vi "Fully Custom Page.vi"(8 "error in (no error)":errorcluster, 11 "Node Ptr":T2 format="%.0x") -> (0 "error out":errorcluster)   [LabVIEW 2011, in "Engine Sim System Explorer.lvlib"]
uses:
  Engine Sim System Explorer.lvlib
  <vilib>/NI Veristand/Custom Device API/Custom Device Item Ref.ctl
  TypeDefs/AngleReference.ctl
  Shared/Engine Simulation Global.vi
  <vilib>/NI Veristand/Custom Device API/Get Item Property (Boolean).vi
  <vilib>/NI Veristand/Custom Device API/Get Item Property (Variant).vi
  <vilib>/NI Veristand/Custom Device API/Get Item Property (U16).vi
  <vilib>/NI Veristand/Custom Device API/Set Item Property (Variant).vi
  <vilib>/NI Veristand/Custom Device API/Set Item Property (Boolean).vi
  <vilib>/Utility/file.llb/Read From Spreadsheet File (DBL).vi
  <vilib>/Utility/file.llb/Write To Spreadsheet File (DBL).vi
  <vilib>/NI Veristand/Custom Device API/Custom Device API.lvlib
  Engine Simulation Shared.lvlib
panel:
  in  "CycleAngle?":T1=TRUE caption="FPGA Simulation Angle Reference"
  in  "Export":bool
  in  "Import":bool
  in  "Tooth Angles":cluster{"Falling Edge":dbl, "Rising Edge":dbl}[](array[cluster])
  in  "SHDocVw.IWebBrowser2":refnum<k7>(container)
  out "N Teeth M Missing View":picture
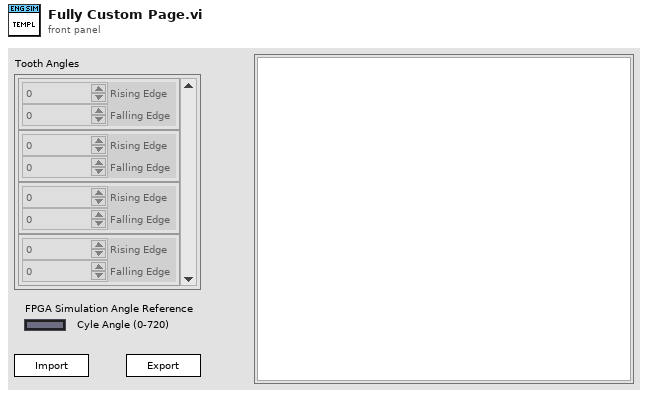
[diagram p1: front panel]
types:
  T1 = typedef "Engine Sim System Explorer.lvlib/AngleReference.ctl" = bool
  T2 = typedef "Custom Device API.lvlib/Custom Device Item Ref.ctl" = u64
  T3 = typedef "Custom Device API.lvlib/Custom Device Commands.ctl" = enum16{"Default", "Item renamed", "Shutdown", "Dynamic button pressed"}
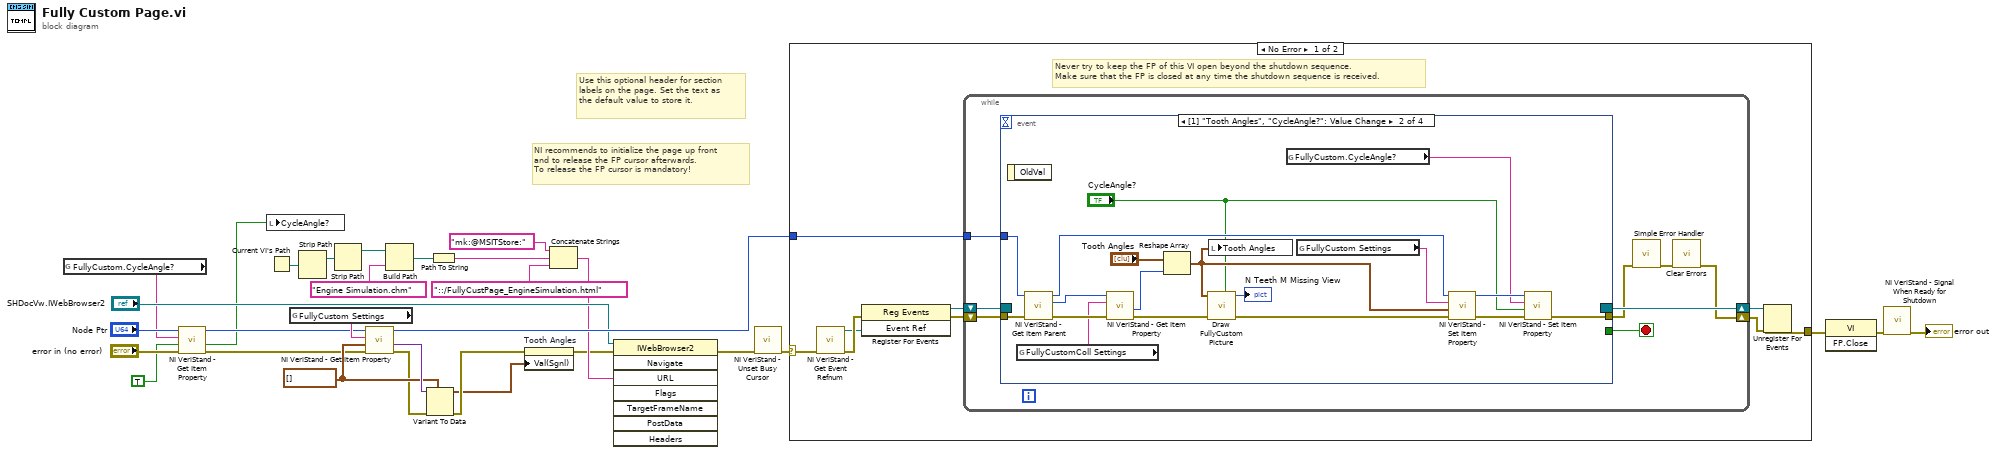
[diagram p0: block diagram]
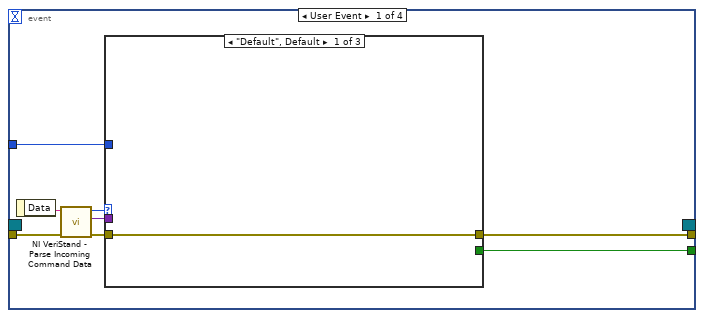
[diagram p2: hidden frame]
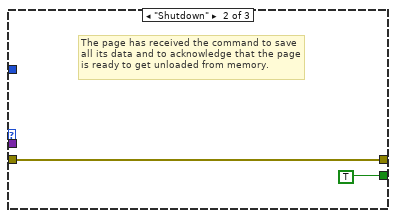
[diagram p3: hidden frame]
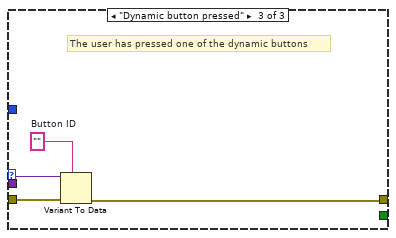
[diagram p4: hidden frame]
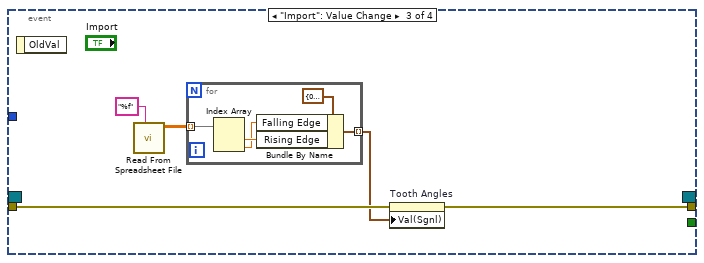
[diagram p5: hidden frame]
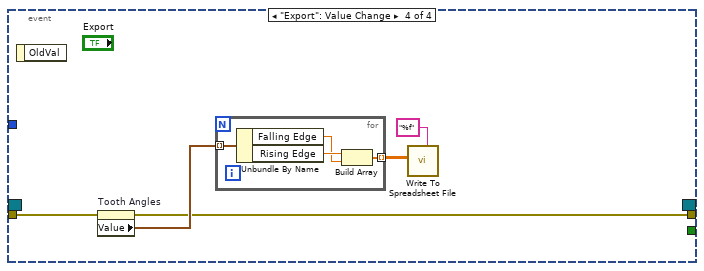
[diagram p6: hidden frame]
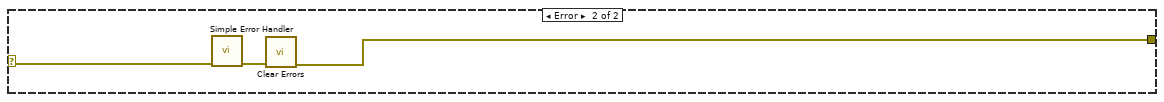
[diagram p7: hidden frame]
diagram:
  w11 = cluster{"Falling Edge":dbl, "Rising Edge":dbl}[] [] ("Tooth Angles")
  # "Use this optional header for section labels on the page. Set the text as the default value to store it."
  # "NI recommends to initialize the page up front\nand to release the FP cursor afterwards.\nTo release the FP cursor is mandatory!"
  n1 = global read "Engine Simulation Global.vi" "FullyCustom.CycleAngle?"() -> (w5:string)
  n2 = call-poly <vilib>:"NI VeriStand - Get Item Property.vi"("error in (no error)"="error in (no error)", "Default Value"=TRUE, "Property Name"=w5, "Item Ref in"="Node Ptr") -> ("error out"=w2:errorcluster, "Value"=w1:bool, "Item Ref out"=w3:T2)  [unwired: 4 in, 1 out]
  n3 = local write "CycleAngle?"(w1) -> ()
  n4 = Current VI's Path() -> (path=w22:path)
  n5 = global read "Engine Simulation Global.vi" "FullyCustom Settings"() -> (w13:string)
  n6 = Strip Path(path=w22) -> (stripped path=w21:path)  [unwired: 1 out]
  n7 = Strip Path(path=w21) -> (stripped path=w16:path)  [unwired: 1 out]
  n8 = call-poly <vilib>:"NI VeriStand - Get Item Property.vi"("error in (no error)"=w2, "Default Value"=w11, "Property Name"=w13, "Item Ref in"=w3) -> ("error out"=w10:errorcluster, "Value"=w12:variant, "Item Ref out"=w25:T2)  [unwired: 4 in, 1 out]
  n9 = Build Path(base path=w16, name or relative path="Engine Simulation.chm") -> (appended path=w18:path)
  n10 = Variant To Data(error in=w10, type=w11, Variant=w12) -> (data=w8:cluster{"Falling Edge":dbl, "Rising Edge":dbl}[], error out=w9:errorcluster)
  n11 = Path To String(path=w18) -> (string=w19:string)
  n12 = property on="Tooth Angles" class="Arr (strict)"(error in=w9, "Val(Sgnl)"=w8) -> (error out=w14:errorcluster)  [unwired: 1 in, 1 out]
  n13 = Concatenate Strings("mk:@MSITStore:" ("string"), w19, "::/FullyCustPage_EngineSimulation.html" ("name or relative path")) -> (w15:string)
  n14 = invoke class="IWebBrowser2" method="Navigate"(reference="SHDocVw.IWebBrowser2", error in=w14, "URL"=w15) -> (error out=w27:errorcluster)  [unwired: 5 in, 7 out]
  n15 = call <vilib>:"NI VeriStand - Unset Busy Cursor.vi"("error in (no error)"=w27) -> ("error out"=w26:errorcluster)  [unwired: 10 out]
  n16 = case shown="No Error" w26 {
    selector: w26 -> [w31 w102]
    tunnel: [w36 w100] -> w30
    tunnel: w25 -> [w32 _]
    frame No Error {
      # "Never try to keep the FP of this VI open beyond the shutdown sequence.\nMake sure that the FP is closed at any time the shutdown sequence is received."
      n17 = call <vilib>:"NI VeriStand - Get Event Refnum.vi"("error in (no error)"=w31) -> ("error out"=w39:errorcluster, "Event Ref"=w35:refnum<user-event>)  [unwired: 9 out]
      n18 = register-events(error in=w39, w35) -> (reference out=w33:refnum<event-registration>, error out=w34:errorcluster)  [unwired: 1 in]
      n19 = while {
        tunnel: w32 -> [w43]
        shift-right: [w40] -> w37
        shift-left: w34 -> [w46]
        shift-right: [w47] -> w38
        shift-left: w33 -> [w45]
        stop <- w44 stop-if-true
        n20 = event shown="[1] \"Tooth Angles\", \"CycleAngle?\": Value Change" {
          selector: w45 -> [_ _ _ _]
          dyn-events: [_ _ _ _] -> w47
          timeout: _ -> [_ _ _ _]
          tunnel: w46 -> [w55 w75 w83 w95]
          tunnel: [w51 _ _ _] -> w44
          tunnel: [w50 w65 w82 w93] -> w42
          tunnel: w43 -> [w49 w74 _ _]
          event User Event {
            n21 = event-data() -> ("Data"=w54:string)  [unwired: 1 out]
            n22 = call <vilib>:"NI VeriStand - Parse Incoming Command Data.vi"("error in (no error)"=w55, "Incoming data"=w54) -> ("error out"=w53:errorcluster, "Outgoing data"=w48:variant, "Action"=w52:T3)  [unwired: 7 out]
            n23 = case shown="\"Default\", Default" w52 {
              tunnel: w53 -> [w56 w57 w62]
              tunnel: [_ TRUE _] -> w51
              tunnel: [w56 w57 w59] -> w50
              tunnel: w49 -> [_ _ _]
              tunnel: w48 -> [_ _ w61]
              frame "Default", Default {
              }
              frame "Shutdown" {
                # "The page has received the command to save all its data and to acknowledge that the page is ready to get unloaded from memory."
              }
              frame "Dynamic button pressed" {
                w60 = ""  # Button ID
                # "The user has pressed one of the dynamic buttons"
                n24 = Variant To Data(error in=w62, type=w60, Variant=w61) -> (error out=w59:errorcluster)  [unwired: 1 out]
              }
            }
          }
          event "Tooth Angles": Value Change {
            n25 = event-data() -> ()  [unwired: 2 out]
            n26 = global read "Engine Simulation Global.vi" "FullyCustomColl Settings"() -> (w69:string)
            n27 = call <vilib>:"NI VeriStand - Get Item Parent.vi"("error in (no error)"=w75, "Item Ref in"=w74) -> ("error out"=w72:errorcluster, "Parent Ref"=w70:T2, "Item Ref out"=w73:T2)  [unwired: 6 in, 1 out]
            n28 = call-poly <vilib>:"NI VeriStand - Get Item Property.vi"("error in (no error)"=w72, "Property Name"=w69, "Item Ref in"=w70) -> ("error out"=w71:errorcluster, "Value"=w68:u16)  [unwired: 5 in, 2 out]
            n29 = Reshape Array("Tooth Angles", w68) -> (w76:cluster{"Falling Edge":dbl, "Rising Edge":dbl}[])
            n30 = call "Draw FullyCustom Picture.vi"("CycleAngle?"="CycleAngle?", "error in (no error)"=w71, "Tooth Angles"=w76) -> ("error out"=w79:errorcluster, "N Teeth M Missing View"=→"N Teeth M Missing View":picture)  [unwired: 7 in]
            n31 = local write "Tooth Angles"(w76) -> ()
            n32 = global read "Engine Simulation Global.vi" "FullyCustom.CycleAngle?"() -> (w64:string)
            n33 = global read "Engine Simulation Global.vi" "FullyCustom Settings"() -> (w78:string)
            n34 = call-poly <vilib>:"NI VeriStand - Set Item Property.vi"("error in (no error)"=w79, "Value"=w76, "Property Name"=w78, "Item Ref in"=w73) -> ("error out"=w66:errorcluster, "Item Ref out"=w67:T2)  [unwired: 5 in, 1 out]
            n35 = call-poly <vilib>:"NI VeriStand - Set Item Property.vi"("error in (no error)"=w66, "Value"="CycleAngle?", "Property Name"=w64, "Item Ref in"=w67) -> ("error out"=w65:errorcluster)  [unwired: 5 in, 2 out]
          }
          event "Import": Value Change {
            n36 = event-data() -> ()  [unwired: 2 out]
            n37 = call-poly <vilib>:"Read From Spreadsheet File.vi"("format (%.3f)"="%f") -> ("all rows"=w84:dbl[][])  [unwired: 6 in, 4 out]
            n38 = for {
              tunnel: w84 -> [w89] mode=indexing
              tunnel: [w86] -> w81 mode=indexing
              n39 = Index Array(array=w89) -> (element #1=w88:dbl, element #2=w87:dbl)  [unwired: 2 in]
              n40 = Bundle By Name(cluster=cluster{"Falling Edge":dbl, "Rising Edge":dbl} {"Falling Edge"=0.0, "Rising Edge"=0.0} ("Tooth"), "Falling Edge"=w87, "Rising Edge"=w88) -> (w86:cluster{"Falling Edge":dbl, "Rising Edge":dbl})
            }
            n41 = property on="Tooth Angles" class="Arr (strict)"(error in=w83, "Val(Sgnl)"=w81) -> (error out=w82:errorcluster)  [unwired: 1 in, 1 out]
          }
          event "Export": Value Change {
            n42 = event-data() -> ()  [unwired: 2 out]
            n43 = property on="Tooth Angles" class="Arr (strict)"(error in=w95) -> (error out=w93:errorcluster, "Value"=w94:cluster{"Falling Edge":dbl, "Rising Edge":dbl}[])  [unwired: 1 in, 1 out]
            n44 = for {
              tunnel: w94 -> [w99] mode=indexing
              tunnel: [w96] -> w92 mode=indexing
              n45 = Unbundle By Name(w99) -> ("Falling Edge"=w97:dbl, "Rising Edge"=w98:dbl)
              n46 = Build Array(w98, w97) -> (w96:dbl[])
            }
            n47 = call-poly <vilib>:"Write To Spreadsheet File.vi"("format (%.3f)"="%f", "2D data"=w92) -> ()  [unwired: 6 in, 1 out]
          }
        }
        n48 = call <vilib>:"Simple Error Handler.vi"("error in (no error)"=w42) -> ("error out"=w41:errorcluster)  [unwired: 1 in, 7 out]
        n49 = call <vilib>:"Clear Errors.vi"("error in (no error)"=w41) -> ("error out"=w40:errorcluster)  [unwired: 6 out]
      }
      n50 = Unregister For Events(event registration refnum=w38, error in=w37) -> (error out=w36:errorcluster)
    }
    frame Error {
      n51 = call <vilib>:"Simple Error Handler.vi"("error in (no error)"=w102) -> ("error out"=w101:errorcluster)  [unwired: 1 in, 7 out]
      n52 = call <vilib>:"Clear Errors.vi"("error in (no error)"=w101) -> ("error out"=w100:errorcluster)  [unwired: 6 out]
    }
  }
  n53 = invoke class="VI" method="FP.Close"(error in=w30) -> (error out=w29:errorcluster)  [unwired: 2 in, 2 out]
  n54 = call <vilib>:"NI VeriStand - Signal When Ready for Shutdown.vi"("error in (no error)"=w29) -> ("error out"=→"error out":errorcluster)  [unwired: 10 out]
